vi "Write Build Time Output Directory.vi"(8 "error in (no error)":errorcluster, 10 "Build Time Output Directory":path, 11 "NSIS Installer in":refnum<class "NSIS Installer.lvclass">) -> (0 "error out":errorcluster, 3 "NSIS Installer out":refnum<class "NSIS Installer.lvclass">)   [LabVIEW 2017, in "CL_G3_VIComponentBuilder.lvlib" / "NSIS Installer.lvclass"]
uses:
  NSIS Installer.lvclass
  NSIS Installer.lvclass/NSIS Installer.ctl
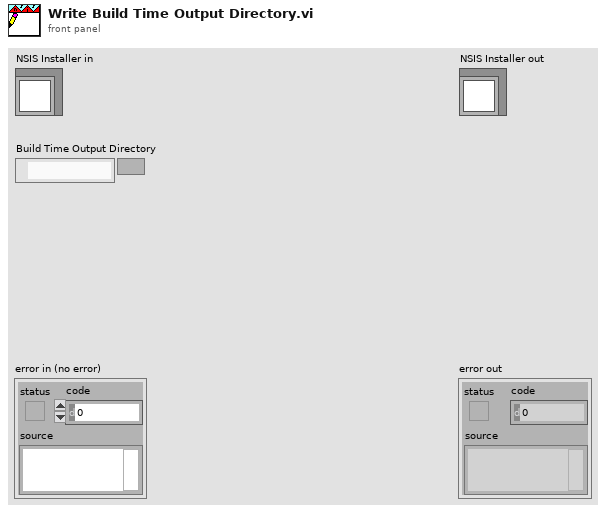
[diagram p1: front panel]
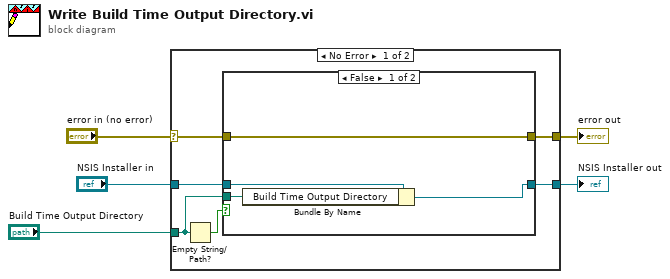
[diagram p0: block diagram]
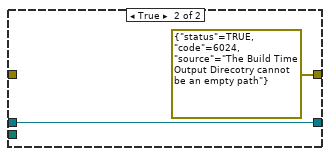
[diagram p2: hidden frame]
diagram:
  n1 = case shown="No Error" "error in (no error)" {
    selector: "error in (no error)" -> [w7 w18]
    tunnel: [w6 w18] -> w4
    tunnel: [w10 w19] -> w2
    tunnel: "NSIS Installer in" -> [w11 w19]
    tunnel: "Build Time Output Directory" -> [w9 _]
    frame No Error {
      n2 = Empty String/Path?(string/path=w9) -> (empty?=w8:bool)
      n3 = case shown="False" w8 {
        tunnel: w11 -> [w15 w17]
        tunnel: [w14 w17] -> w10
        tunnel: w9 -> [w13 _]
        tunnel: w7 -> [w12 _]
        tunnel: [w12 errorcluster {"status"=TRUE, "code"=6024, "source"="The Build Time Output Direcotry cannot be an empty path"} ("error in (no error)")] -> w6
        frame False {
          n4 = Bundle By Name(cluster=w15, "Build Time Output Directory"=w13) -> (w14:refnum<class "NSIS Installer.lvclass">)
        }
        frame True {
        }
      }
    }
    frame Error {
    }
  }
  "error out" <- w4
  "NSIS Installer out" <- w2
